vi "getMirRotMat.vi"(8 "error in (no error)":errorcluster, 10 "Rotation Angle in Deg":dbl, 11 "CamRot in":refnum<class "CamRot.lvclass">) -> (0 "error out":errorcluster, 2 "Rotation Matrix":dbl[][](array[numeric]), 3 "CamRot out":refnum<class "CamRot.lvclass">)   [LabVIEW 2016, in "CamRot.lvclass"]
doc: "Get the mirror rotation matrix."
uses:
  CamRot.lvclass
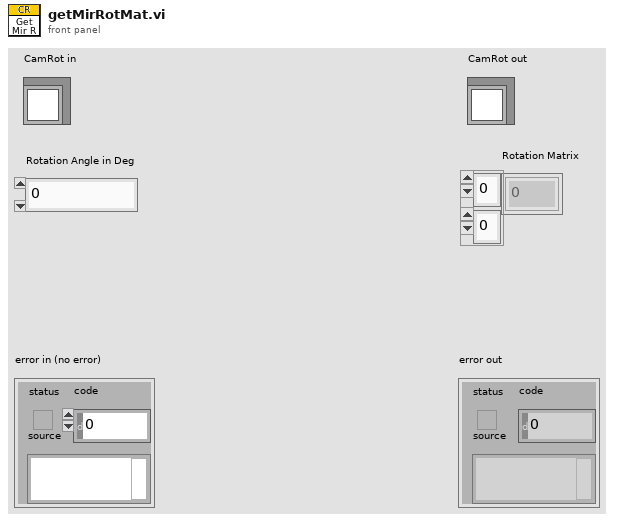
[diagram p1: front panel]
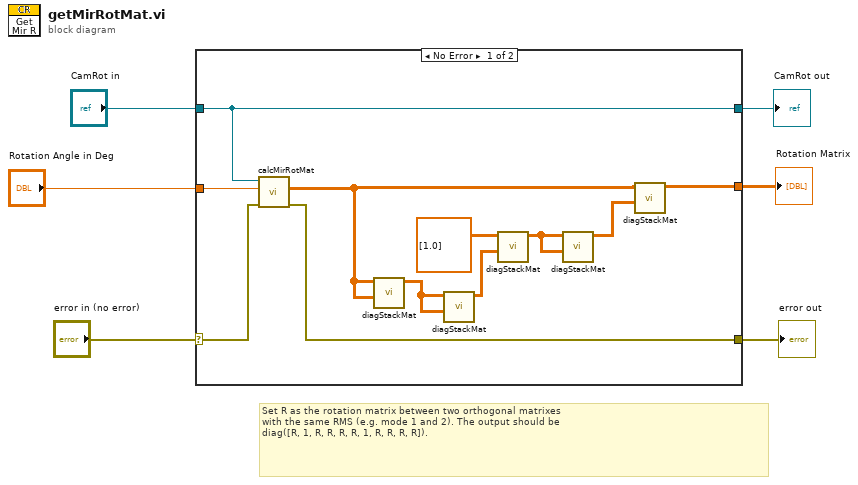
[diagram p0: block diagram]
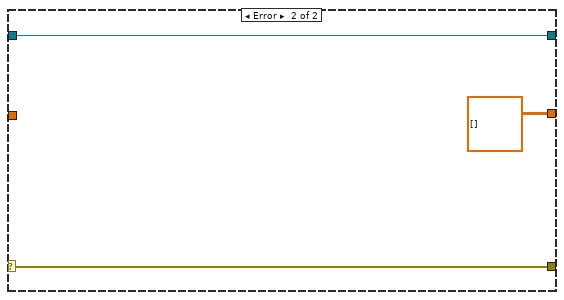
[diagram p2: hidden frame]
diagram:
  # "Set R as the rotation matrix between two orthogonal matrixes\nwith the same RMS (e.g. mode 1 and 2). The output should be\ndiag([R, 1, R, R, R, R, 1, R, R, R, R])."
  n1 = case shown="No Error" "error in (no error)" {
    selector: "error in (no error)" -> [w16 w20]
    tunnel: [w15 w20] -> w5
    tunnel: [w17 w19] -> w3
    tunnel: "CamRot in" -> [w17 w19]
    tunnel: "Rotation Angle in Deg" -> [w14 _]
    tunnel: [w7 dbl[][] [] ("Diag Stack Matrix")] -> w1
    frame No Error {
      n2 = call "calcMirRotMat.vi"("error in (no error)"=w16, "Rotation Angle in Deg"=w14, "CamRot in"=w17) -> ("error out"=w15:errorcluster, "Rotation Matrix"=w9:dbl[][])  [unwired: 6 in, 1 out]
      n3 = call "diagStackMat.vi"("A1"=w9, "A0"=w9) -> ("Diag Stack Matrix"=w13:dbl[][])  [unwired: 9 in]
      n4 = call "diagStackMat.vi"("A1"=w13, "A0"=w13) -> ("Diag Stack Matrix"=w11:dbl[][])  [unwired: 9 in]
      n5 = call "diagStackMat.vi"("A1"=w11, "A0"=dbl[][] [[1.0]]) -> ("Diag Stack Matrix"=w10:dbl[][])  [unwired: 9 in]
      n6 = call "diagStackMat.vi"("A1"=w10, "A0"=w10) -> ("Diag Stack Matrix"=w8:dbl[][])  [unwired: 9 in]
      n7 = call "diagStackMat.vi"("A1"=w8, "A0"=w9) -> ("Diag Stack Matrix"=w7:dbl[][])  [unwired: 9 in]
    }
    frame Error {
    }
  }
  "error out" <- w5
  "CamRot out" <- w3
  "Rotation Matrix" <- w1
